vi "LAB8A.vi"() -> ()   [LabVIEW 2018]
panel:
  in  "FUNCTION":sgl(slide) scale=0.0..3.0
  out "ANSWER":dbl
  in  "#2":dbl
  in  "#1":dbl
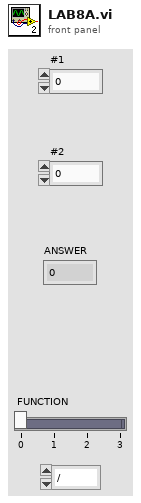
[diagram p1: front panel]
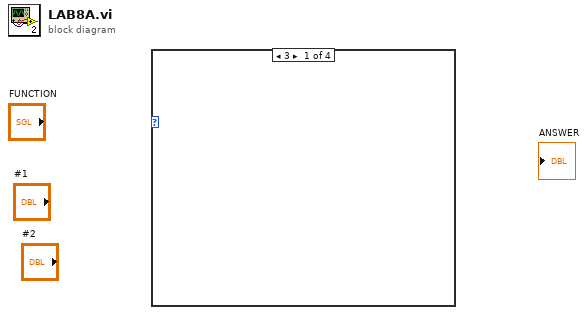
[diagram p0: block diagram]
diagram:
  n1 = case shown="3" {
    selector: _ -> [_ _ _ _]
    frame 3 {
    }
    frame 2 {
    }
    frame 1 {
    }
    frame 0 {
    }
  }
